vi "ReportLoopTime.vi"(11 "NT_Name":string) -> ()   [LabVIEW 2023]
uses:
  <vilib>/Rock Robotics/WPI/ThirdParty/JAS_Junk/TrajLib/Trajectory_Library.lvlib
  <vilib>/Rock Robotics/WPI/ThirdParty/JAS_Junk/TrajLib/LinearFilter_MovingAvg_Execute.vi
  <vilib>/Rock Robotics/Network Tables/NT Write Number.vi
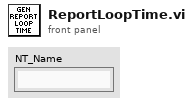
[diagram p1: front panel]
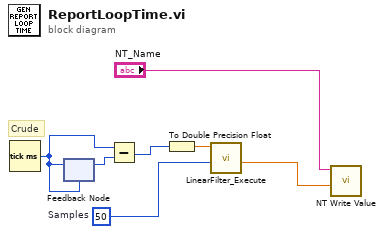
[diagram p0: block diagram]
diagram:
  w3 = 50  # Samples
  # "Crude"
  n1 = Tick Count (ms)() -> (millisecond timer value=w2:u32)
  n2 = feedback #1(w2) -> (w1:u32)
  n3 = feedback-in #1(w2) -> ()
  n4 = Subtract(x=w2, y=w1) -> (x-y=w5:u32)
  n5 = To Double Precision Float(number=w5) -> (double precision float=w4:dbl)
  n6 = call-poly <vilib>:"LinearFilter_Execute.vi"("Samples"=w3, "Input"=w4) -> ("Output"=w6:dbl)  [unwired: 9 in]
  n7 = call-poly <vilib>:"NT Write Value.vi"("value"=w6, "name"="NT_Name") -> ()  [unwired: 9 in, 1 out]
